vi "Get Main Pane.vi"(8 "error in":errorcluster, 11 "Flex UI in":refnum<class "Flex UI.lvclass">) -> (0 "error out":errorcluster, 3 "Flex UI out":refnum<class "Flex UI.lvclass">)   [LabVIEW 2016, in "Flex UI.lvclass"]
uses:
  Flex UI.lvclass
  Flex UI.lvclass/Flex UI.ctl
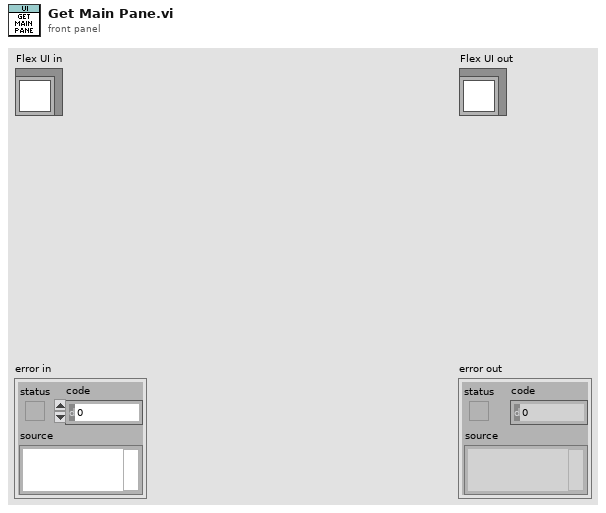
[diagram p1: front panel]
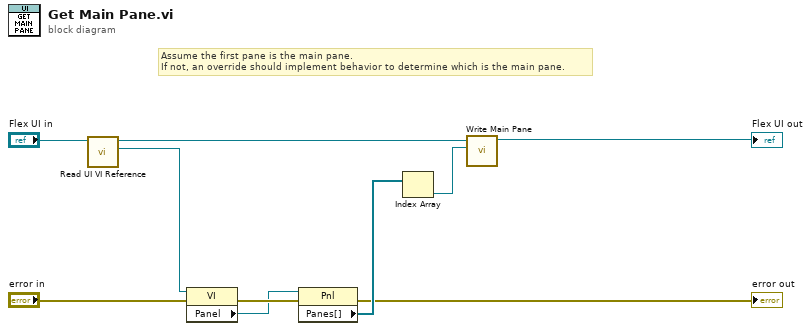
[diagram p0: block diagram]
diagram:
  # "Assume the first pane is the main pane.\nIf not, an override should implement behavior to determine which is the main pane."
  n1 = call "Read UI VI Reference.vi"("Flex UI in"="Flex UI in") -> ("UI VI Reference"=w3:refnum<vi>, "Flex UI out"=w4:refnum<class "Flex UI.lvclass">)  [unwired: 9 in]
  n2 = property class="VI"(reference=w3, error in="error in") -> (error out=w10:errorcluster, "Panel"=w2:refnum<vi>)  [unwired: 1 out]
  n3 = property class="Pnl"(reference=w2, error in=w10) -> (error out=→"error out":errorcluster, "Panes[]"=w8:refnum<vi>[])  [unwired: 1 out]
  n4 = Index Array(array=w8) -> (element=w9:refnum<vi>)  [unwired: 1 in]
  n5 = call "Write Main Pane.vi"("Main Pane"=w9, "Flex UI in"=w4) -> ("Flex UI out"=→"Flex UI out":refnum<class "Flex UI.lvclass">)  [unwired: 9 in]
